vi "VCS Enable Position Window.vi"(8 "error in (no error)":errorcluster, 10 "position window":T1, 11 "axis in":cluster{"keyHandle":u32, "nodeId":u16}={"keyHandle"=0, "nodeId"=1}) -> (0 "error out":errorcluster, 3 "axis out":cluster{"keyHandle":u32, "nodeId":u16}={"keyHandle"=0, "nodeId"=1})   [LabVIEW 2017, in "maxonEPOS.lvlib"]
doc: "With function <B>VCS_EnablePositionWindow</B> the position window is activated."
uses:
  Examples/maxonEPOS.lvlib
  SSI_Tool/InstrumentsInterfaces/Motordriver/maxon EPOS/Resources/EposCmd.dll
  SSI_Tool/InstrumentsInterfaces/Motordriver/maxon EPOS/Resources/EposCmd64.dll
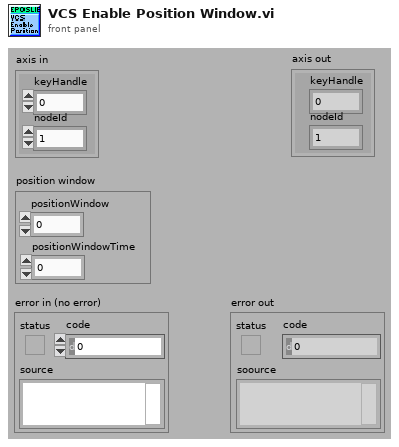
[diagram p1: front panel]
types:
  T1 = cluster{"positionWindow":u32, "positionWindowTime":u16}
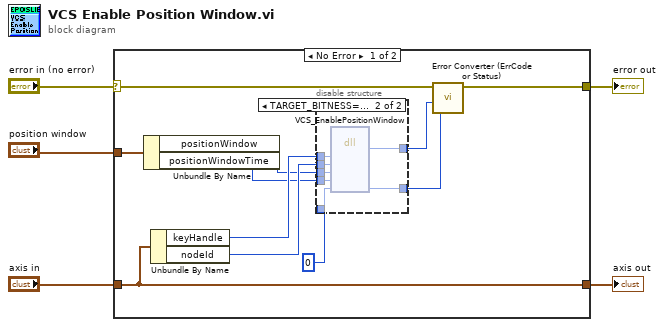
[diagram p0: block diagram]
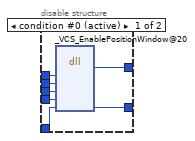
[diagram p2: hidden frame]
diagram:
  n1 = case shown="No Error" "error in (no error)" {
    selector: "error in (no error)" -> [w14 w31]
    tunnel: "axis in" -> [w16 w32]
    tunnel: [w16 w32] -> w4
    tunnel: [w15 w31] -> w3
    tunnel: "position window" -> [w8 _]
    frame No Error {
      n2 = Unbundle By Name(w8) -> ("positionWindow"=w6:u32, "positionWindowTime"=w7:u16)
      n3 = Unbundle By Name(w16) -> ("keyHandle"=w10:u32, "nodeId"=w9:u16)
      n4 = disable-structure shown="TARGET_BITNESS==64" {
        disable-tunnel: u32 0 ("pErrorCode") -> [w23 w30]
        disable-tunnel: [w22 w29] -> w12
        disable-tunnel: [w21 w28] -> w11
        disable-tunnel: w10 -> [w20 w27]
        disable-tunnel: w9 -> [w19 w26]
        disable-tunnel: w7 -> [w18 w25]
        disable-tunnel: w6 -> [w17 w24]
        frame condition #0 (active) {
          n5 = dll-call lib="C:/workspace/project/scancon/sw/SSI_Tool/InstrumentsInterfaces/Motordriver/maxon EPOS/Resources/EposCmd.*" fn="_VCS_EnablePositionWindow@20"("KeyHandle"=w20, "NodeId"=w19, "PositionWindow"=w17, "PositionWindowTime"=w18, "pErrorCode"=w23) -> (w21:i32, "pErrorCode"=w22:u32)  [unwired: 7 in, 2 out]
        }
        frame condition #1 {
          n6 = dll-call lib="C:/setup/Resources/EposCmd64.*" fn="VCS_EnablePositionWindow" ("EposCmd.dll:_VCS_EnablePositionWindow@20")("KeyHandle"=w27, "NodeId"=w26, "PositionWindow"=w24, "PositionWindowTime"=w25, "pErrorCode"=w30) -> ("Rückgabetyp"=w28:i32, "pErrorCode"=w29:u32)  [unwired: 7 in, 2 out]
        }
      }
      n7 = call "Error Converter (ErrCode or Status).vi"("error code"=w12, "return type"=w11, "error in (no error)"=w14) -> ("error out"=w15:errorcluster)  [unwired: 7 in]
    }
    frame Error {
    }
  }
  "error out" <- w3
  "axis out" <- w4
